vi "milliGAT Configure and Run Continuous - Parallel.vi"() -> ()   [LabVIEW 2015]
uses:
  Global FIA milliGAT.lvlib
  Public/Utility/Pump Direction.ctl
  Public/Utility/Pump Address.ctl
panel:
  out "error out closing":errorcluster
  in  "Flow Parameters 2":T1={"Peak Flow (uL/s)"=1.0, "Starting Flow (uL/s)"=0.1, "Acceleration (uL/s^2)"=500.0, "Deceleration (uL/s^2)"=500.0}
  in  "Pump ID (0:A) 2":T2=enum."B"
  in  "Stop 2":bool
  out "Microliters 2":dbl
  in  "Direction 2":T3=enum."Dispense"
  in  "Serial Configuration 2":cluster{"Baud Rate":u32}={"Baud Rate"=9600} {"Baud Rate" items=["300"=300, "600"=600, "1200"=1200, "2400"=2400, "4800"=4800, "9600"=9600, "19200"=19200]}
  out "error out 2":errorcluster
  in  "Flow Parameters":T1={"Peak Flow (uL/s)"=0.5, "Starting Flow (uL/s)"=0.1, "Acceleration (uL/s^2)"=500.0, "Deceleration (uL/s^2)"=500.0}
  in  "Pump ID (0:A)":T2
  in  "Stop":bool
  out "Microliters":dbl
  in  "Direction":T3=enum."Dispense"
  in  "Serial Configuration":cluster{"Baud Rate":u32}={"Baud Rate"=9600} {"Baud Rate" items=["300"=300, "600"=600, "1200"=1200, "2400"=2400, "4800"=4800, "9600"=9600, "19200"=19200]}
  out "error out":errorcluster
  in  "VISA resource name":refnum<visa-resource-name>="COM16"
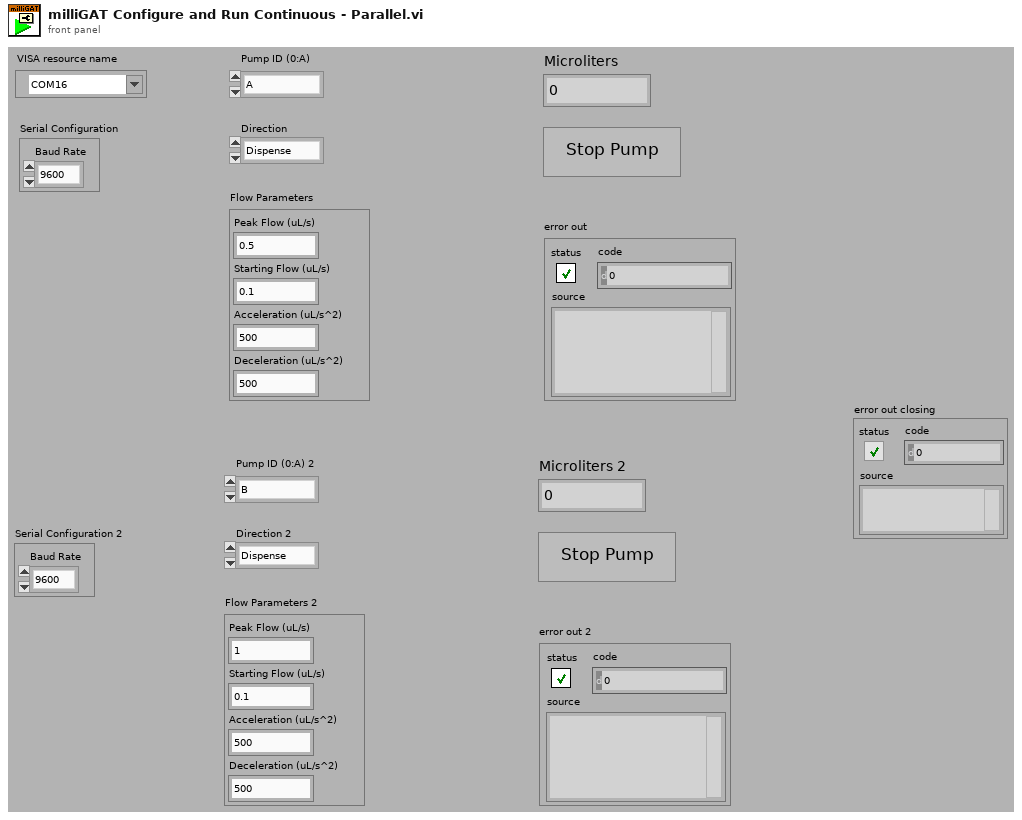
[diagram p1: front panel]
types:
  T1 = cluster{"Peak Flow (uL/s)":dbl, "Starting Flow (uL/s)":dbl, "Acceleration (uL/s^2)":dbl, "Deceleration (uL/s^2)":dbl}
  T2 = typedef "Global FIA milliGAT.lvlib/Pump Address.ctl" = enum16{"A", "B", "C", "D", "E", "F", "G", "H", "I", "J", "K", "L", "M", "N", "O", "P", "Q", "R", "S", "T", "U", "V", "W", "X", "Y", "Z", "a", "b", "c", "d", "e", "f", "g", "h", "i", "j", "k", "l", "m", "n", "o", "p", "q", "r", "s", "t", "u", "v", "w", "x", "y", "z", "0", "1", "2", "3", "4", "5", "6", "7", "8", "9"}
  T3 = typedef "Global FIA milliGAT.lvlib/Pump Direction.ctl" = enum16{"Aspirate", "Dispense"}
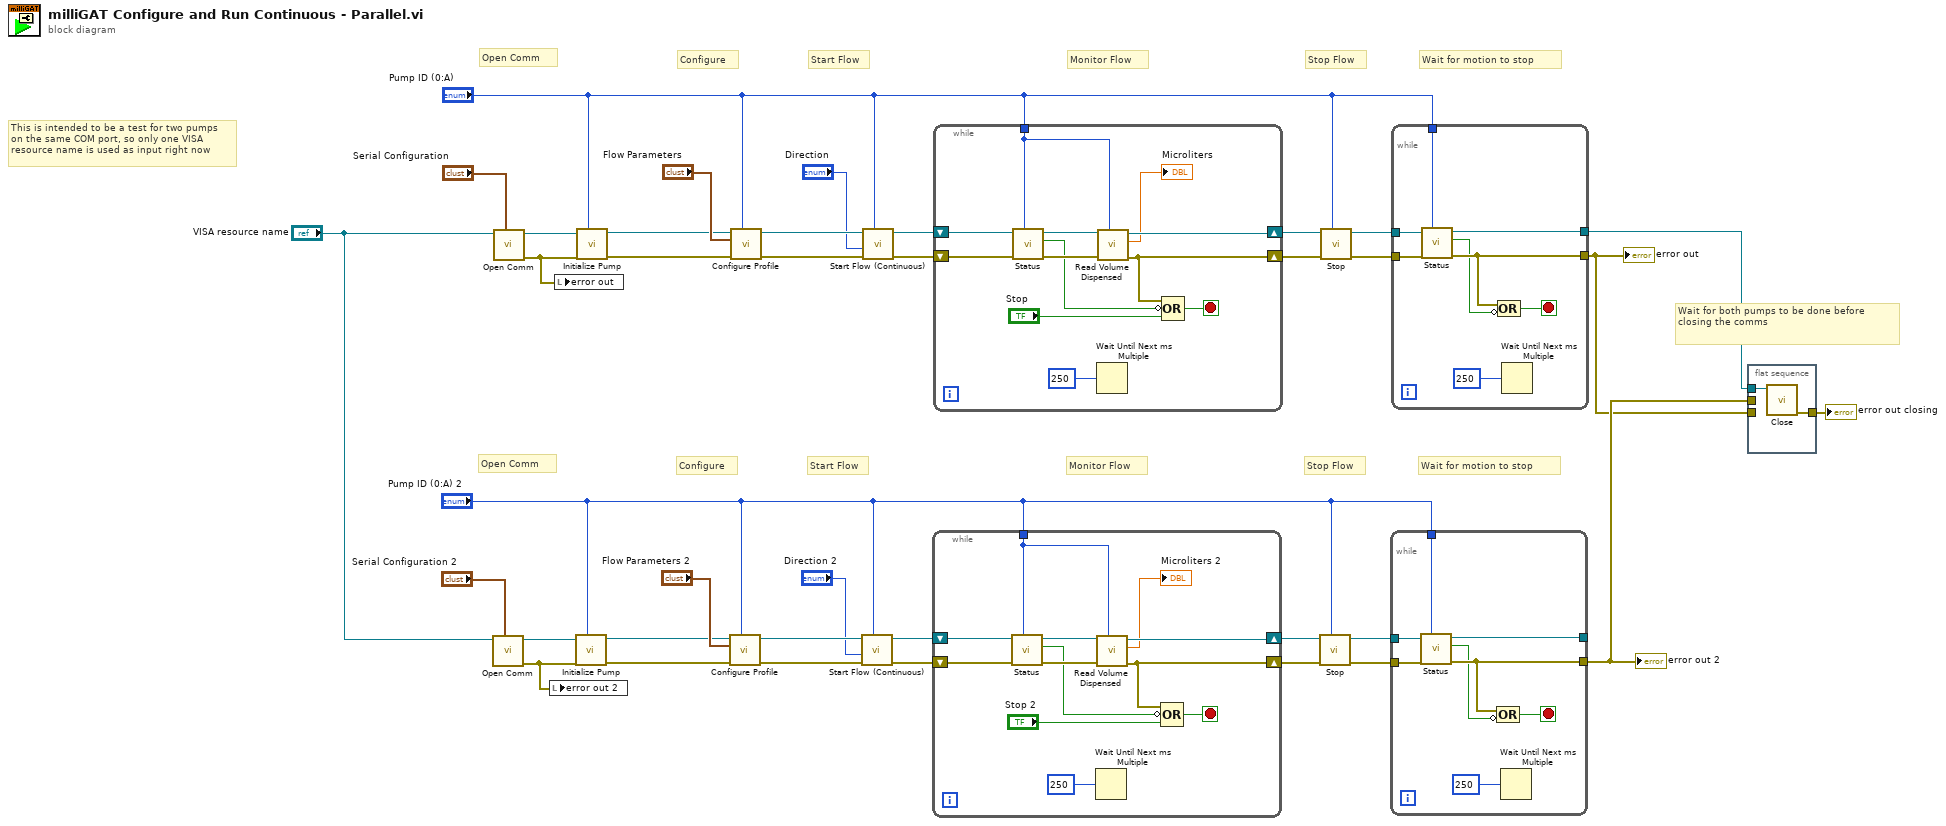
[diagram p0: block diagram]
diagram:
  # "This is intended to be a test for two pumps\non the same COM port, so only one VISA\nresource name is used as input right now"
  # "Wait for both pumps to be done before closing the comms"
  # "Stop Flow"
  # "Open Comm"
  # "Start Flow"
  # "Configure"
  # "Monitor Flow"
  # "Wait for motion to stop"
  # "Stop Flow"
  # "Open Comm"
  # "Start Flow"
  # "Configure"
  # "Monitor Flow"
  # "Wait for motion to stop"
  n1 = call "Open Comm.vi"("Serial Configuration"="Serial Configuration 2", "VISA resource in"="VISA resource name") -> ("error out"=w8:errorcluster, "VISA resource out"=w14:refnum<visa-resource-name>)  [unwired: 8 in]
  n2 = call "Open Comm.vi"("Serial Configuration"="Serial Configuration", "VISA resource in"="VISA resource name") -> ("error out"=w24:errorcluster, "VISA resource out"=w31:refnum<visa-resource-name>)  [unwired: 8 in]
  n3 = local write "error out 2"(w8) -> ()
  n4 = local write "error out"(w24) -> ()
  n5 = call "Initialize Pump.vi"("Pump ID (0:A)"="Pump ID (0:A) 2", "error in (no error)"=w8, "VISA resource in"=w14) -> ("error out"=w5:errorcluster, "VISA resource out"=w6:refnum<visa-resource-name>)  [unwired: 7 in]
  n6 = call "Initialize Pump.vi"("Pump ID (0:A)"="Pump ID (0:A)", "error in (no error)"=w24, "VISA resource in"=w31) -> ("error out"=w21:errorcluster, "VISA resource out"=w22:refnum<visa-resource-name>)  [unwired: 7 in]
  n7 = call "Configure Profile.vi"("Pump ID (0:A)"="Pump ID (0:A) 2", "error in (no error)"=w5, "Flow Parameters"="Flow Parameters 2", "VISA resource in"=w6) -> ("error out"=w19:errorcluster, "VISA resource out"=w20:refnum<visa-resource-name>)  [unwired: 6 in]
  n8 = call "Configure Profile.vi"("Pump ID (0:A)"="Pump ID (0:A)", "error in (no error)"=w21, "Flow Parameters"="Flow Parameters", "VISA resource in"=w22) -> ("error out"=w36:errorcluster, "VISA resource out"=w37:refnum<visa-resource-name>)  [unwired: 6 in]
  n9 = call "Start Flow (Continuous).vi"("Pump ID (0:A)"="Pump ID (0:A) 2", "error in (no error)"=w19, "Direction (0:Aspirate)"="Direction 2", "VISA resource in"=w20) -> ("error out"=w16:errorcluster, "VISA resource out"=w17:refnum<visa-resource-name>)  [unwired: 6 in]
  n10 = call "Start Flow (Continuous).vi"("Pump ID (0:A)"="Pump ID (0:A)", "error in (no error)"=w36, "Direction (0:Aspirate)"="Direction", "VISA resource in"=w37) -> ("error out"=w33:errorcluster, "VISA resource out"=w34:refnum<visa-resource-name>)  [unwired: 6 in]
  n11 = while {
    shift-right: [w49] -> w11
    shift-left: w17 -> [w47]
    tunnel: "Pump ID (0:A) 2" -> [w46]
    shift-right: [w39] -> w12
    shift-left: w16 -> [w48]
    stop <- w41 stop-if-true
    n12 = call "Status.vi"("Pump ID (0:A)"=w46, "error in (no error)"=w48, "VISA resource in"=w47) -> ("error out"=w43:errorcluster, "moving"=w38:bool, "VISA resource out"=w44:refnum<visa-resource-name>)  [unwired: 6 in]
    n13 = Wait Until Next ms Multiple(millisecond multiple=u32 250) -> ()  [unwired: 1 out]
    n14 = call "Read Volume Dispensed.vi"("Pump ID (0:A)"=w46, "error in (no error)"=w43, "VISA resource in"=w44) -> ("error out"=w39:errorcluster, "microliters"=→"Microliters 2":dbl, "VISA resource out"=w49:refnum<visa-resource-name>)  [unwired: 6 in]
    n15 = Compound Arithmetic op=OR(w39, invert w38, "Stop 2") -> (w41:bool)
  }
  n16 = while {
    shift-right: [w61] -> w28
    shift-left: w34 -> [w59]
    tunnel: "Pump ID (0:A)" -> [w58]
    shift-right: [w51] -> w29
    shift-left: w33 -> [w60]
    stop <- w53 stop-if-true
    n17 = call "Status.vi"("Pump ID (0:A)"=w58, "error in (no error)"=w60, "VISA resource in"=w59) -> ("error out"=w55:errorcluster, "moving"=w50:bool, "VISA resource out"=w56:refnum<visa-resource-name>)  [unwired: 6 in]
    n18 = Wait Until Next ms Multiple(millisecond multiple=u32 250) -> ()  [unwired: 1 out]
    n19 = call "Read Volume Dispensed.vi"("Pump ID (0:A)"=w58, "error in (no error)"=w55, "VISA resource in"=w56) -> ("error out"=w51:errorcluster, "microliters"=→"Microliters":dbl, "VISA resource out"=w61:refnum<visa-resource-name>)  [unwired: 6 in]
    n20 = Compound Arithmetic op=OR(w51, invert w50, "Stop") -> (w53:bool)
  }
  n21 = call "Stop.vi"("Pump ID (0:A)"="Pump ID (0:A) 2", "error in (no error)"=w12, "VISA resource in"=w11) -> ("error out"=w10:errorcluster, "VISA resource out"=w9:refnum<visa-resource-name>)  [unwired: 7 in]
  n22 = call "Stop.vi"("Pump ID (0:A)"="Pump ID (0:A)", "error in (no error)"=w29, "VISA resource in"=w28) -> ("error out"=w27:errorcluster, "VISA resource out"=w26:refnum<visa-resource-name>)  [unwired: 7 in]
  n23 = while {
    tunnel: w10 -> [w68]
    tunnel: w9 -> [w69]
    tunnel: "Pump ID (0:A) 2" -> [w67]
    tunnel: [w65] -> w3
    tunnel: [w66] -> _
    stop <- w63 stop-if-true
    n24 = call "Status.vi"("Pump ID (0:A)"=w67, "error in (no error)"=w68, "VISA resource in"=w69) -> ("error out"=w65:errorcluster, "moving"=w64:bool, "VISA resource out"=w66:refnum<visa-resource-name>)  [unwired: 6 in]
    n25 = Compound Arithmetic op=OR(w65, invert w64) -> (w63:bool)
    n26 = Wait Until Next ms Multiple(millisecond multiple=u32 250) -> ()  [unwired: 1 out]
  }
  "error out 2" <- w3
  n27 = while {
    tunnel: w27 -> [w76]
    tunnel: w26 -> [w77]
    tunnel: "Pump ID (0:A)" -> [w75]
    tunnel: [w73] -> w2
    tunnel: [w74] -> w25
    stop <- w71 stop-if-true
    n28 = call "Status.vi"("Pump ID (0:A)"=w75, "error in (no error)"=w76, "VISA resource in"=w77) -> ("error out"=w73:errorcluster, "moving"=w72:bool, "VISA resource out"=w74:refnum<visa-resource-name>)  [unwired: 6 in]
    n29 = Compound Arithmetic op=OR(w73, invert w72) -> (w71:bool)
    n30 = Wait Until Next ms Multiple(millisecond multiple=u32 250) -> ()  [unwired: 1 out]
  }
  "error out" <- w2
  n31 = flat-sequence {
    tunnel: w25 -> [w79]
    tunnel: w3 -> [_]
    tunnel: w2 -> [_]
    tunnel: [w78] -> w1
    frame #0 {
      n32 = call "Close.vi"("VISA resource in"=w79) -> ("error out"=w78:errorcluster)  [unwired: 10 in]
    }
  }
  "error out closing" <- w1
